vi "Stop.vi"(8 "error in (no error)":errorcluster, 11 "NI SMU in":refnum<class "NI SMU.lvclass">) -> (0 "error out":errorcluster, 3 "NI SMU out":refnum<class "NI SMU.lvclass">)   [LabVIEW 2020, in "NI SMU.lvlib" / "NI SMU.lvclass"]
uses:
  NI SMU.lvclass
  NI SMU.lvclass/NI SMU.ctl
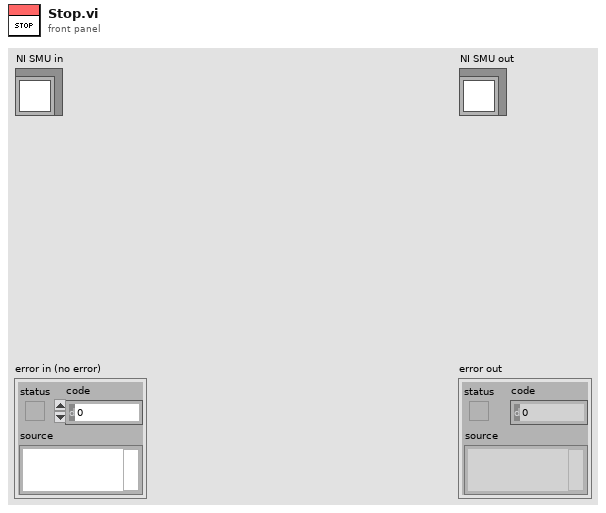
[diagram p1: front panel]
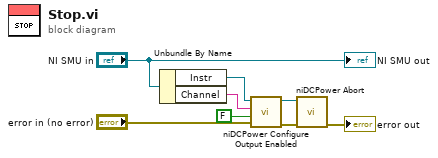
[diagram p0: block diagram]
diagram:
  n1 = Unbundle By Name("NI SMU in") -> ("Instr"=w4:refnum<k15>, "Channel"=w3:string)
  n2 = call <instrlib>:"niDCPower Configure Output Enabled.vi"("error in (no error)"="error in (no error)", "output enabled"=FALSE, "channel name"=w3, "instrument handle"=w4) -> ("error out"=w6:errorcluster, "instrument handle out"=w7:refnum<k15>)  [unwired: 6 in]
  n3 = call <instrlib>:"niDCPower Abort.vi"("error in (no error)"=w6, "instrument handle"=w7) -> ("error out"=→"error out":errorcluster)  [unwired: 8 in, 1 out]
  "NI SMU out" <- "NI SMU in"
